vi "test2.vi"() -> ()   [LabVIEW 2015]
uses:
  APP/excelFile_class/fileType.ctl
  APP/excelFile_class/excelFile.lvclass
panel:
  in  "Path":path
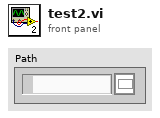
[diagram p1: front panel]
types:
  T1 = typedef "excelFile.lvclass/fileType.ctl" = enum16{"database", "CosmedTest"}
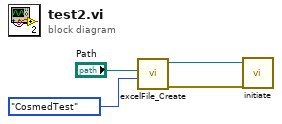
[diagram p0: block diagram]
diagram:
  n1 = call "excelFile_Create.vi"("fileType"=fileType."CosmedTest", "Path"="Path") -> ("error out"=w1:errorcluster, "reference out"=w4:refnum<class "excelFile.lvclass">)  [unwired: 8 in]
  n2 = call-dynamic "initiate.vi"("reference in"=w4, "error in (no error)"=w1) -> ()  [unwired: 16 in, 2 out]
